vi "Get_STREAM_TYPE.vi"(5 "Device Number":T2, 7 "Update":bool, 11 "Protocol (in)":T1=enum."SPI") -> (3 "Protocol (out)":T1=enum."SPI")   [LabVIEW 2016]
uses:
  _TypeDefs/FRIC_navX_DeviceNumbersTypeDef.ctl
  _TypeDefs/Z900_navX_ProtocolTypeDef.ctl
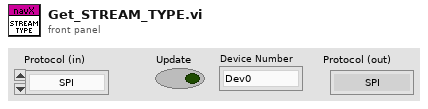
[diagram p1: front panel]
types:
  T1 = typedef "Z900_navX_ProtocolTypeDef.ctl" = enum16{"SERIAL", "I2C", "SPI"}
  T2 = typedef "FRIC_navX_DeviceNumbersTypeDef.ctl" = enum16{"Dev0", "Dev1", "Dev2", "Dev3"}
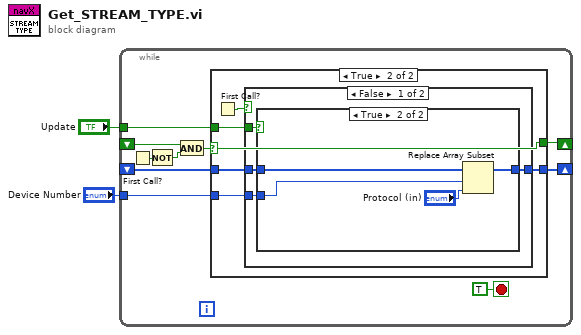
[diagram p0: block diagram]
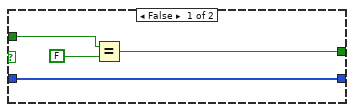
[diagram p2: hidden frame]
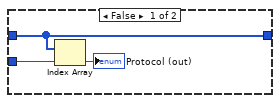
[diagram p3: hidden frame]
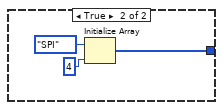
[diagram p4: hidden frame]
diagram:
  n1 = while {
    shift-right: [w12] -> _
    shift-left: _ -> [w9]
    tunnel: "Update" -> [w10]
    tunnel: "Device Number" -> [w8]
    shift-right: [w3] -> _
    shift-left: _ -> [w5]
    stop <- TRUE stop-if-true
    n2 = First Call?() -> (First Call?: T/F=w6:bool)
    n3 = Not(x=w6) -> (.not. x?=w7:bool)
    n4 = And(x=w5, y=w7) -> (x .and. y?=w4:bool)
    n5 = case shown="True" w4 {
      selector: w4 -> [_ w17]
      tunnel: [w16 w22] -> w12
      tunnel: w10 -> [w14 w21]
      tunnel: w9 -> [w16 w20]
      tunnel: w8 -> [_ w19]
      tunnel: [w13 w17] -> w3
      frame False {
        n6 = Equal?(x=w14, y=FALSE) -> (x = y?=w13:bool)
      }
      frame True {
        n7 = First Call?() -> (First Call?: T/F=w18:bool)
        n8 = case shown="False" w18 {
          tunnel: [w26 w36] -> w22
          tunnel: w21 -> [w25 _]
          tunnel: w20 -> [w24 _]
          tunnel: w19 -> [w23 _]
          frame False {
            n9 = case shown="True" w25 {
              tunnel: [w29 w32] -> w26
              tunnel: w24 -> [w29 w33]
              tunnel: w23 -> [w28 w31]
              frame False {
                n10 = Index Array(array=w29, index=w28) -> (element=→"Protocol (out)":T1)
              }
              frame True {
                n11 = Replace Array Subset(array=w33, new element="Protocol (in)", index=w31) -> (w32:T1[])
              }
            }
          }
          frame True {
            n12 = Initialize Array(Z900_navX_ProtocolTypeDef."SPI" ("Protocol (in)"), 4 ("dimension size")) -> (w36:T1[])
          }
        }
      }
    }
  }
